vi "Time calculation.vi"(0 "2nd sample":i16, 1 "3rd sample":i16, 3 "2nd sample":i16, 4 "3rd sample":i16, 5 "4th sample":i16, 6 "5th sample":i16, 8 "4th sample":i16, 9 "5th sample":i16) -> (7 "Time between first and last waveform":ext format="%#.7g")   [LabVIEW 2012]
panel:
  out "seconds":ext
  out "Time in min":ext
  out "time in s for the last waveform":ext
  out "timing in samples last waveform":u64
  out "time in s for the first waveform":ext
  out "hi(x) 3":i16
  out "lo(x) 3":i16
  out "hi(x) 4":i16
  out "lo(x) 4":i16
  out "timing in samples":u64
  # "Input"
  # "Input time of last waveform"
  # "Crosscheck"
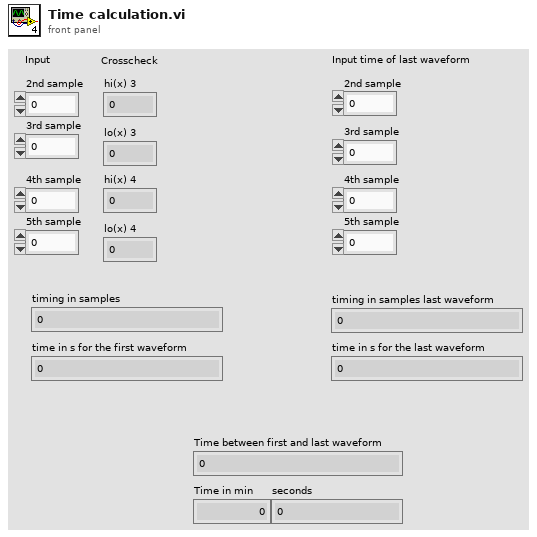
[diagram p1: front panel]
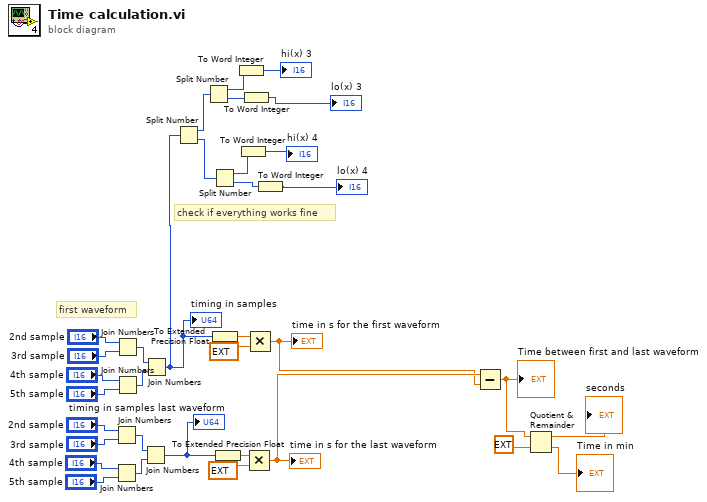
[diagram p0: block diagram]
diagram:
  # "first waveform"
  # "check if everything works fine"
  n1 = Join Numbers(hi="2nd sample", lo="3rd sample") -> ((hi.lo)=w16:u32)
  n2 = Join Numbers(hi="4th sample", lo="5th sample") -> ((hi.lo)=w17:u32)
  n3 = Join Numbers(hi="2nd sample", lo="3rd sample") -> ((hi.lo)=w30:u32)
  n4 = Join Numbers(hi="4th sample", lo="5th sample") -> ((hi.lo)=w29:u32)
  n5 = Join Numbers(hi=w16, lo=w17) -> ((hi.lo)=w13:u64)
  "timing in samples last waveform" <- w13
  n6 = Join Numbers(hi=w30, lo=w29) -> ((hi.lo)=w5:u64)
  "timing in samples" <- w5
  n7 = Split Number(x=w5) -> (hi(x)=w27:u32, lo(x)=w28:u32)
  n8 = Split Number(x=w27) -> (hi(x)=w26:u16, lo(x)=w24:u16)
  n9 = Split Number(x=w28) -> (hi(x)=w22:u16, lo(x)=w20:u16)
  n10 = To Extended Precision Float(1:w5) -> (0:w10:ext)
  n11 = To Extended Precision Float(1:w13) -> (0:w9:ext)
  n12 = To Word Integer(number=w26) -> (16bit integer=→"hi(x) 3":i16)
  n13 = To Word Integer(number=w22) -> (16bit integer=→"hi(x) 4":i16)
  n14 = To Word Integer(number=w24) -> (16bit integer=→"lo(x) 3":i16)
  n15 = Multiply(x=w9, y=ext 2e-8) -> (x*y=w12:ext)
  "time in s for the last waveform" <- w12
  n16 = Multiply(x=w10, y=ext 2e-8) -> (x*y=w11:ext)
  "time in s for the first waveform" <- w11
  n17 = To Word Integer(number=w20) -> (16bit integer=→"lo(x) 4":i16)
  n18 = Subtract(x=w12, y=w11) -> (x-y=w4:ext)
  "Time between first and last waveform" <- w4
  n19 = Quotient & Remainder(x=w4, y=ext 60.0) -> (x-y*floor(x/y)=→"seconds":ext, floor(x/y)=→"Time in min":ext)
